vi "choosePath.vi"(8 "error in (no error)":errorcluster, 10 "ImagesTaken":i32, 11 "Pixelfly in":refnum<class "PixelflySA.lvclass">) -> (0 "error out":errorcluster, 2 "Path":path, 3 "Pixelfly out":refnum<class "PixelflySA.lvclass">)   [LabVIEW 2011, in "PixelflySA.lvclass"]
uses:
  PixelflySA.lvclass
  PixelflySA.lvclass/PixelflySA.ctl
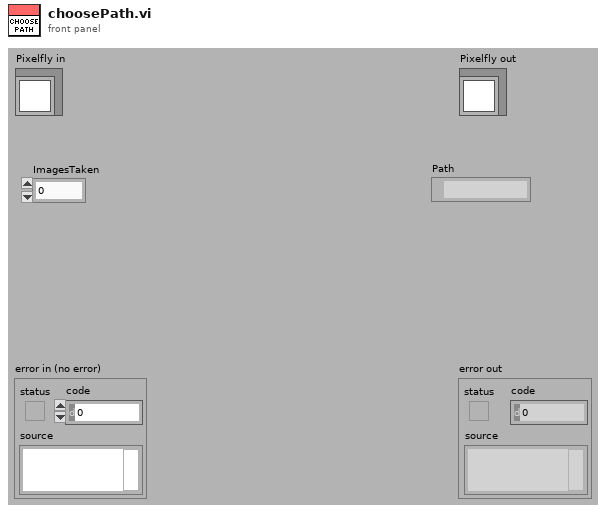
[diagram p1: front panel]
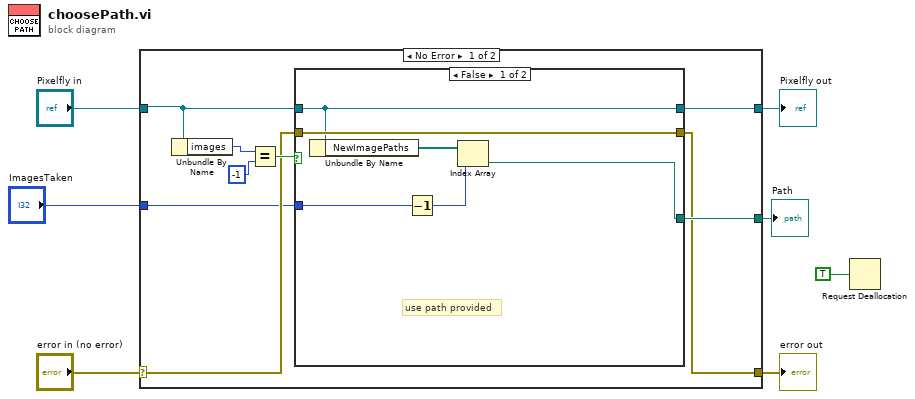
[diagram p0: block diagram]
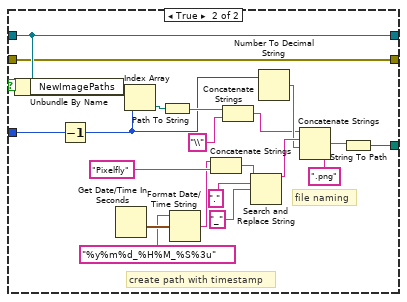
[diagram p2: hidden frame]
diagram:
  n1 = case shown="No Error" "error in (no error)" {
    selector: "error in (no error)" -> [w11 w45]
    tunnel: [w9 w45] -> w6
    tunnel: [w15 w44] -> w4
    tunnel: "Pixelfly in" -> [w16 w44]
    tunnel: [w10 _] -> w3
    tunnel: "ImagesTaken" -> [w8 _]
    frame No Error {
      n2 = Unbundle By Name(w16) -> ("images"=w14:i32)
      n3 = Equal?(x=w14, y=-1) -> (x = y?=w12:bool)
      n4 = case shown="False" w12 {
        tunnel: w16 -> [w19 w26]
        tunnel: [w19 w26] -> w15
        tunnel: w11 -> [w20 w25]
        tunnel: [w20 w25] -> w9
        tunnel: [w22 w30] -> w10
        tunnel: w8 -> [w18 w24]
        frame False {
          # "use path provided"
          n5 = Unbundle By Name(w19) -> ("NewImagePaths"=w21:path[])
          n6 = Decrement(x=w18) -> (x-1=w17:i32)
          n7 = Index Array(array=w21, index=w17) -> (element=w22:path)
        }
        frame True {
          # "create path with timestamp"
          # "file naming"
          n8 = Unbundle By Name(w26) -> ("NewImagePaths"=w27:path[])
          n9 = Decrement(x=w24) -> (x-1=w23:i32)
          n10 = Get Date/Time In Seconds() -> (seconds since 1Jan1904=w42:timestamp)
          n11 = Index Array(array=w27, index=w23) -> (element=w28:path)
          n12 = Path To String(path=w28) -> (string=w29:string)
          n13 = Format Date/Time String(time format string (%c)="%y%m%d_%H%M_%S%3u", seconds (now)=w42) -> (date/time string=w40:string)  [unwired: 1 in]
          n14 = Concatenate Strings(w40, "Pixelfly") -> (w39:string)
          n15 = Concatenate Strings(w29, "\\") -> (w32:string)
          n16 = Search and Replace String(input string=w39, search string=".", replace string="_") -> (result string=w35:string)  [unwired: 5 in, 3 out]
          n17 = Number To Decimal String(number=w23) -> (decimal integer string=w34:string)  [unwired: 1 in]
          n18 = Concatenate Strings(w32, w35, w34, ".png") -> (w31:string)
          n19 = String To Path(string=w31) -> (path=w30:path)
        }
      }
    }
    frame Error {
    }
  }
  "error out" <- w6
  "Pixelfly out" <- w4
  "Path" <- w3
  n20 = Request Deallocation(TRUE ("flag")) -> ()
